vi "DisplayResIdErrorZ.vi"(5 "First iteration":bool, 6 "error in (no error)":errorcluster, 7 "warnings in":errorcluster, 8 "measSetId":i32, 9 "measResId":i32) -> (0 "error out":errorcluster, 1 "VI's path":string="InterruptMeasZ.vi", 2 "ID summary":T1(array[cluster]))   [LabVIEW 2016]
doc: "This program displays results of measurements which have already been completed, while further measurements are being run. The measurement setting and result IDs (measSetId and measResId) are displayed along with any errors or warnings found.\n\nWhen the program is called, the input results are added to the previous list, which is maintained using an uninitialized shift register. If the \"First iteration\" input is true, the previous list is cleared."
panel:
  # "Program constants"
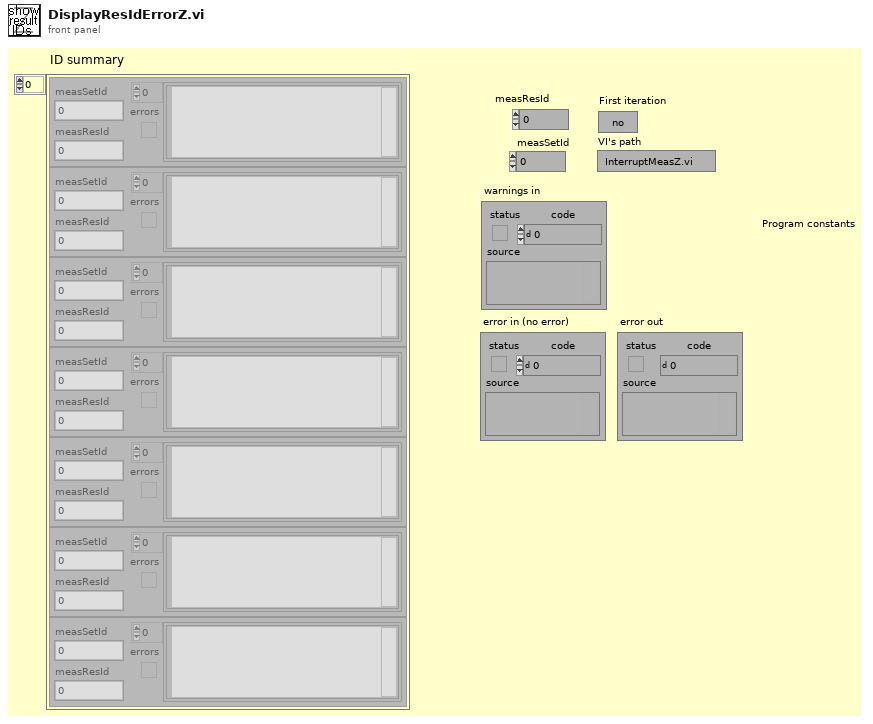
[diagram p1: front panel]
types:
  T1 = cluster{"measSetId":i32, "measResId":i32, "errors":string[], "status":bool}[]
  T2 = cluster{"measSetId":i32, "measResId":i32, "errors":string[], "status":bool}
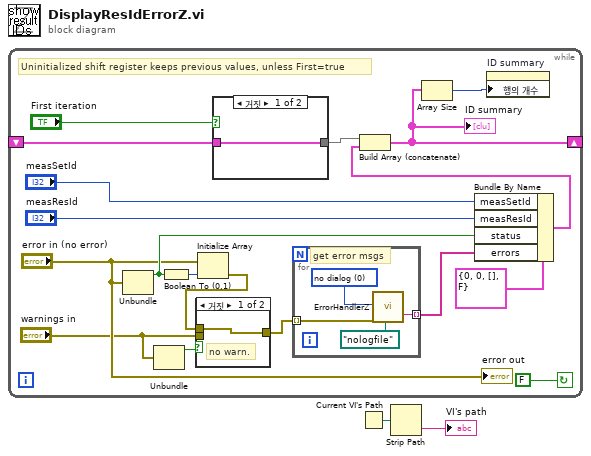
[diagram p0: block diagram]
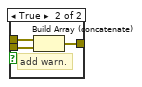
[diagram p2: hidden frame]
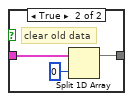
[diagram p3: hidden frame]
diagram:
  n1 = while {
    shift-left: _ -> [w15]
    shift-right: [w12] -> _
    stop <- FALSE continue-if-true
    # "Uninitialized shift register keeps previous values, unless First=true"
    n2 = Unbundle("error in (no error)") -> ("status"=w10:bool)  [unwired: 2 out]
    n3 = Unbundle("warnings in") -> ("status"=w7:bool)  [unwired: 2 out]
    n4 = Boolean To (0,1)(Boolean=w10) -> (0, 1=w8:i16)
    n5 = Initialize Array("error in (no error)", w8) -> (w5:errorcluster[])
    n6 = case shown="거짓" w7 {
      tunnel: "warnings in" -> [_ w23]
      tunnel: w5 -> [w21 w24]
      tunnel: [w21 w22] -> w4
      frame False {
        # "no warn."
      }
      frame True {
        # "add warn."
        n7 = Build Array (concatenate)(w24, w23) -> (w22:errorcluster[])
      }
    }
    n8 = case shown="거짓" "First iteration" {
      tunnel: [w25 w26] -> w16
      tunnel: w15 -> [w25 w28]
      frame False {
      }
      frame True {
        # "clear old data"
        n9 = Split 1D Array(array=w28, index=0) -> (first subarray=w26:T1)  [unwired: 1 out]
      }
    }
    n10 = for {
      tunnel: w4 -> [w32] mode=indexing
      tunnel: [w29] -> w20 mode=indexing
      w31 = u16 0 items=["no dialog", "timed OK message", "timed options message"] ("type of dialog (timed opt:2)")
      # "get error msgs"
      n11 = call "ErrorHandlerZ.vi"("type of dialog (timed opt:2)"=w31, "error in (no error)"=w32, "Log file"=path "nologfile") -> ("message"=w29:string)  [unwired: 11 in, 5 out]
    }
    n12 = Bundle By Name(cluster=T2 {"measSetId"=0, "measResId"=0, "errors"=[], "status"=FALSE} ("Cluster"), "measSetId"="measSetId", "measResId"="measResId", "status"=w10, "errors"=w20) -> (w18:T2)
    n13 = Build Array (concatenate)(w16, w18) -> (w12:T1)
    "ID summary" <- w12
    n14 = Array Size(array=w12) -> (size(s)=w13:i32)
    n15 = property on="ID summary" class="Arr (엄격한)"("행의 개수"=w13) -> ()  [unwired: 2 in, 2 out]
    "error out" <- "error in (no error)"
  }
  n16 = Current VI's Path() -> (path=w1:path)
  n17 = Strip Path(path=w1) -> (name=→"VI's path":string)  [unwired: 1 out]
